vi "Common_Socket_Cmd_Sub_VI_Testmode.vi"(4 "Time Delay":i16=10, 6 "Common Socket Error in":errorcluster, 7 "Response ID 1":u8, 8 "Operation Message Length 1":i32, 9 "Operation Message ID 1":i32, 11 "connection ID":refnum<k5>) -> (0 "Pass":string="Horn Scan Success", 1 "error out":errorcluster, 3 "connection ID":refnum<k5>)   [LabVIEW 2017]
panel:
  out "*(type *) &x":u8
  out "rest of the binary string":string
  out "Test mode Message Length":u8
  out "Test mode Message ID":u8
  out "bytes written":i32
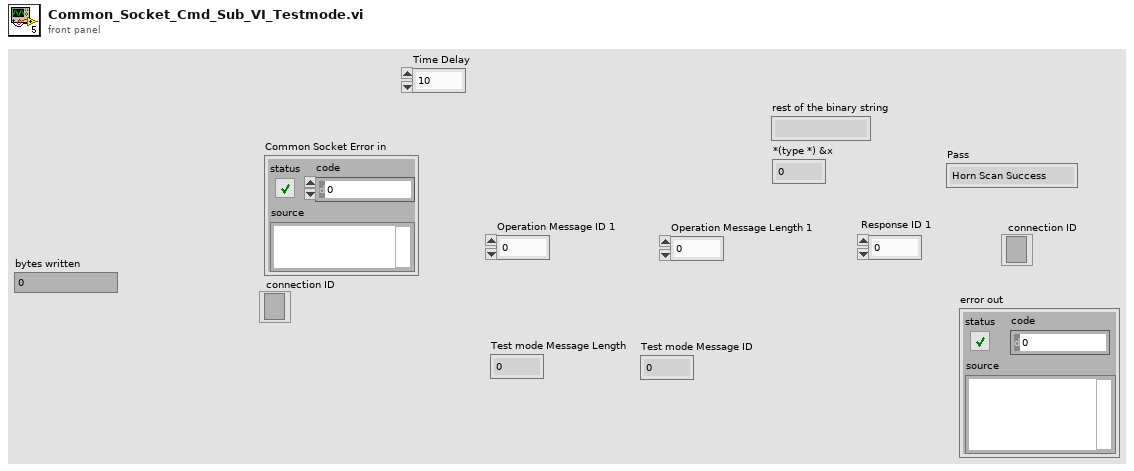
[diagram p1: front panel]
types:
  T1 = enum16{"big-endian, network order", "native, host order", "little-endian"}
  T2 = cluster{"Operation Message Length 1":i32, "Operation Message ID 1":i32}
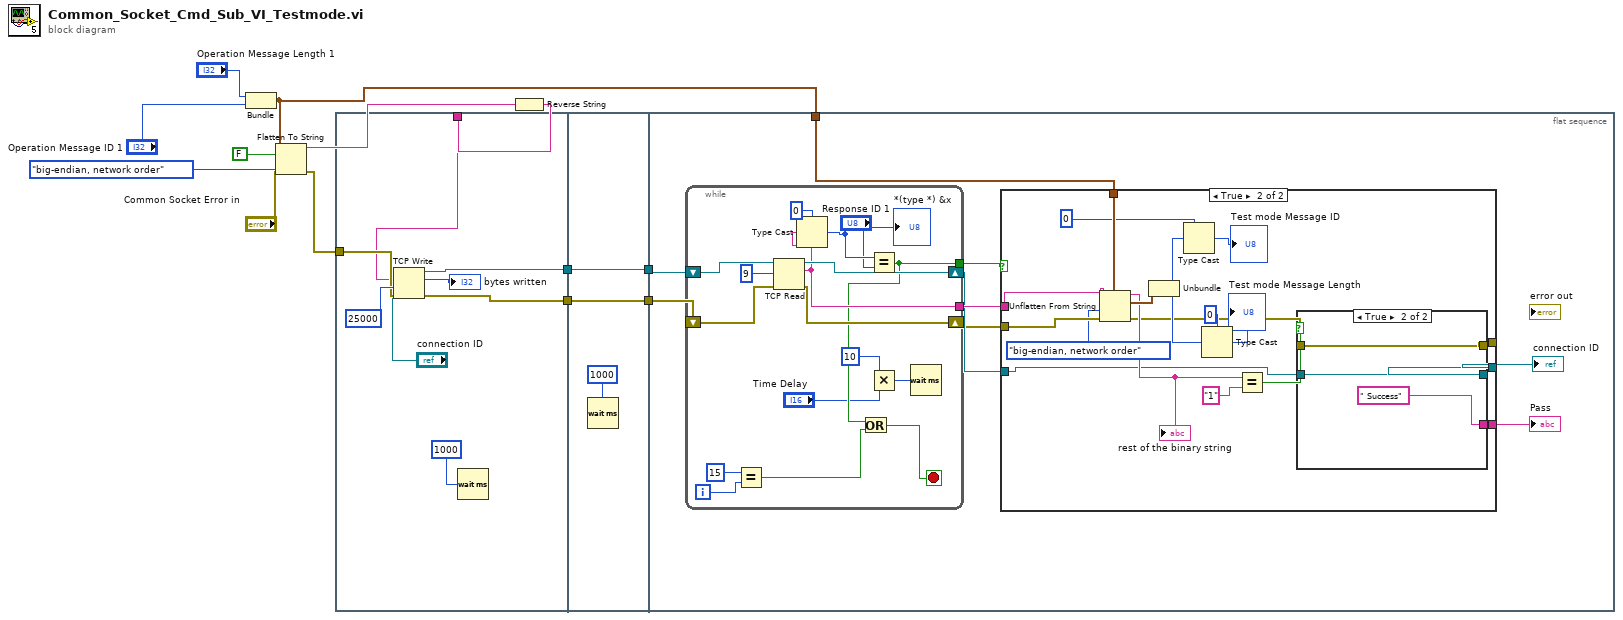
[diagram p0: block diagram]
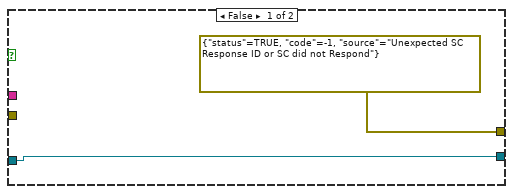
[diagram p2: hidden frame]
diagram:
  n1 = Bundle("Operation Message Length 1"="Operation Message Length 1", "Operation Message ID 1"="Operation Message ID 1") -> (w2:T2)  [unwired: 1 in]
  n2 = Flatten To String(anything=w2, prepend array or string size? (T)=FALSE, byte order (0:big-endian, network order)=T1."big-endian, network order", error in (no error)="Common Socket Error in") -> (data string=w5:string, error out=w6:errorcluster)  [unwired: 1 out]
  n3 = flat-sequence {
    tunnel: [w19] -> w13
    tunnel: [w18] -> w12
    tunnel: w6 -> [w17]
    tunnel: w4 -> [w16]
    tunnel: [w23] -> w11
    tunnel: w13 -> [w23]
    tunnel: [w22] -> w10
    tunnel: w12 -> [w22]
    tunnel: w11 -> [w33]
    tunnel: w10 -> [w32]
    tunnel: w2 -> [w31]
    frame #0 {
      n4 = TCP Write(connection ID="connection ID", data in=w16, error in (no error)=w17, 9:25000 ("timeout ms (25000)")) -> (connection ID out=w19:refnum<k5>, bytes written=→"bytes written":i32, error out=w18:errorcluster)
      n5 = Wait (ms)(milliseconds to wait=u32 1000) -> ()  [unwired: 1 out]
    }
    frame #1 {
      n6 = Wait (ms)(milliseconds to wait=u32 1000) -> ()  [unwired: 1 out]
    }
    frame #2 {
      n7 = while {
        tunnel: [w71] -> w30
        shift-right: [w74] -> w27
        shift-left: w33 -> [w76]
        shift-right: [w72] -> w25
        shift-left: w32 -> [w75]
        tunnel: [w67] -> w29
        i -> [w65]
        stop <- w66 stop-if-true
        n8 = Equal?(x=15, y=w65) -> (x = y?=w63:bool)
        n9 = TCP Read(connection ID=w76, bytes to read=9, error in (no error)=w75) -> (connection ID out=w74:refnum<k5>, data out=w71:string, error out=w72:errorcluster)  [unwired: 2 in]
        n10 = Type Cast(type=u8 0, x=w71) -> (*(type *) &x=w69:u8)
        "*(type *) &x" <- w69
        n11 = Equal?(x=w69, y="Response ID 1") -> (x = y?=w67:bool)
        n12 = Or(x=w67, y=w63) -> (x .or. y?=w66:bool)
        n13 = Multiply(x=i16 10 ("milliseconds to wait"), y="Time Delay") -> (x*y=w61:i16)
        n14 = Wait (ms)(milliseconds to wait=w61) -> ()  [unwired: 1 out]
      }
      n15 = case shown="True" w29 {
        tunnel: w31 -> [_ w53]
        tunnel: w30 -> [_ w46]
        tunnel: w25 -> [_ w45]
        tunnel: [w35 w37] -> w28
        tunnel: w27 -> [w35 w38]
        tunnel: [errorcluster {"status"=TRUE, "code"=-1, "source"="Unexpected SC Response ID or SC did not Respond"} ("error constant") w39] -> _
        tunnel: [_ w36] -> w26
        frame False {
        }
        frame True {
          n16 = Unflatten From String(type=w53, binary string=w46, byte order (0:big-endian, network order)=T1."big-endian, network order", error in (no error)=w45) -> (rest of the binary string=w43:string, value=w54:T2, error out=w40:errorcluster)  [unwired: 1 in]
          "rest of the binary string" <- w43
          n17 = Unbundle(w54) -> ("Operation Message Length 1"=w48:i32, "Operation Message ID 1"=w52:i32)
          n18 = Type Cast(type=u8 0, x=w48) -> (*(type *) &x=→"Test mode Message ID":u8)
          n19 = Type Cast(type=u8 0, x=w52) -> (*(type *) &x=→"Test mode Message Length":u8)
          n20 = Equal?(x=w43, y="1") -> (x = y?=w41:bool)
          n21 = case shown="True" w41 {
            tunnel: w40 -> [w55 w59]
            tunnel: [w55 w59] -> w39
            tunnel: w38 -> [w56 w58]
            tunnel: [w56 w58] -> w37
            tunnel: [_ " Success"] -> w36
            frame False {
            }
            frame True {
            }
          }
        }
      }
      "connection ID" <- w28
      "Pass" <- w26
    }
  }
  n22 = Reverse String(1:w5) -> (0:w4:string)
